vi "TransistorOnOff.vi"() -> ()   [LabVIEW 2014]
uses:
  <vilib>/DAQmx/create/channels.llb/DAQmx Create Channel (AI-Voltage-Basic).vi
  <vilib>/DAQmx/create/channels.llb/DAQmx Create Channel (DO-Digital Output).vi
  <vilib>/DAQmx/read.llb/DAQmx Read (Analog DBL 1Chan 1Samp).vi
  <vilib>/DAQmx/write.llb/DAQmx Write (Digital Bool 1Line 1Point).vi
panel:
  out "?":bool
  in  "VREF \nVoltage Measured from unheated":dbl
  out "Analog Voltage":dbl
  in  "Ambient Temperature (C)":dbl=22.0
  in  "Low Setpoint (C)":dbl=30.0
  in  "Hi Setpoint (C)":dbl=33.0
  in  "dt (ms)":dbl=0.5 format="%#_13g"
  out "Sample Temp":dbl
  out "?":dbl(graph)
  in  "?":bool
  out "Heater Output":dbl(slide) scale=0.0..1.0
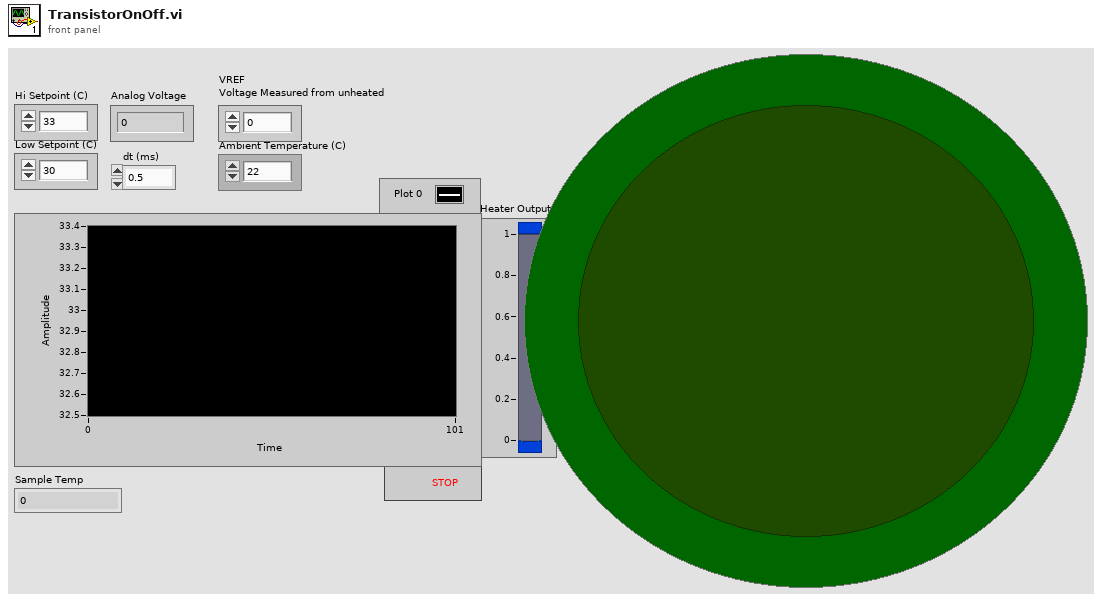
[diagram p1: front panel]
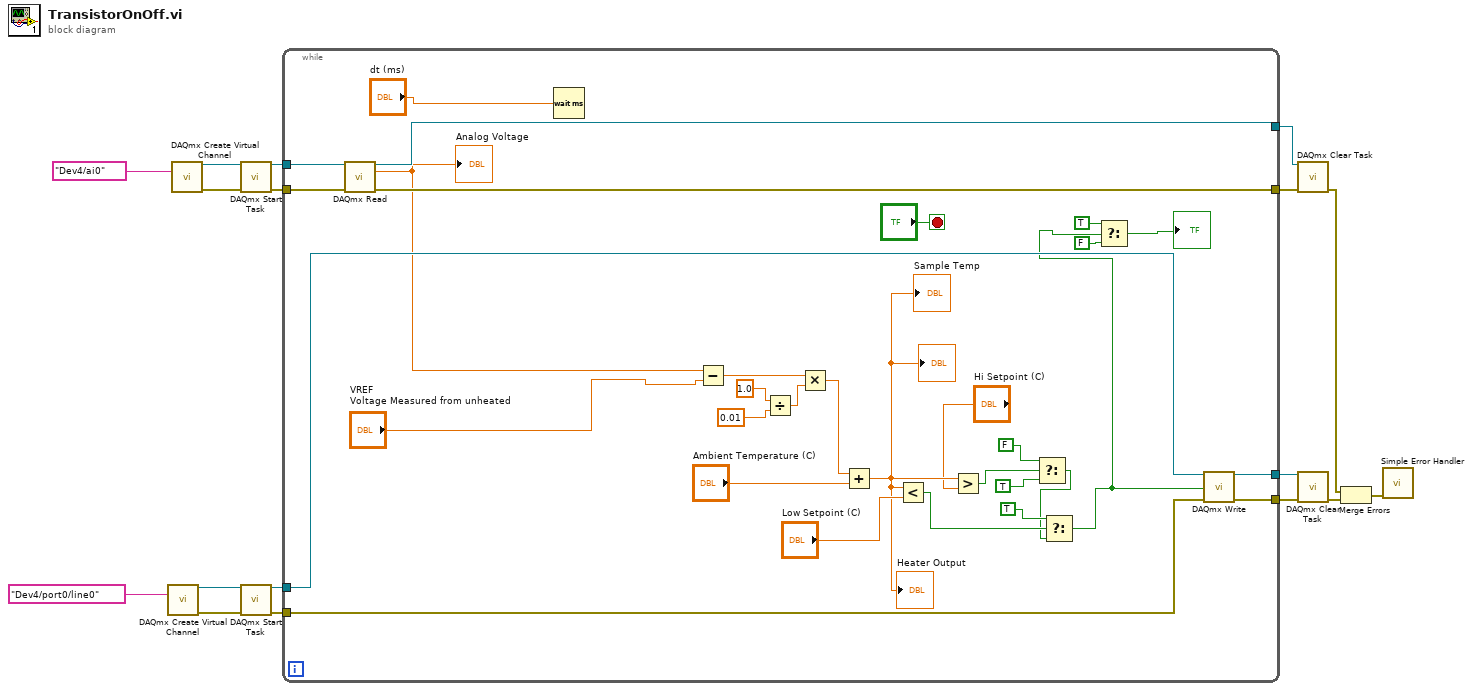
[diagram p0: block diagram]
diagram:
  n1 = call-poly <vilib>:"DAQmx Create Virtual Channel.vi"("lines"=tag "Dev4/port0/line0") -> ("task out"=w10:refnum<k21>, "error out"=w9:errorcluster)  [unwired: 13 in]
  n2 = call-poly <vilib>:"DAQmx Create Virtual Channel.vi"("physical channels"=tag "Dev4/ai0") -> ("task out"=w16:refnum<k21>, "error out"=w17:errorcluster)  [unwired: 13 in]
  n3 = call <vilib>:"DAQmx Start Task.vi"("task/channels in"=w16, "error in"=w17) -> ("task out"=w14:refnum<k21>, "error out"=w13:errorcluster)  [unwired: 12 in]
  n4 = call <vilib>:"DAQmx Start Task.vi"("task/channels in"=w10, "error in"=w9) -> ("task out"=w8:refnum<k21>, "error out"=w7:errorcluster)  [unwired: 12 in]
  n5 = while {
    tunnel: w14 -> [w47]
    tunnel: w13 -> [w46]
    tunnel: [w45] -> w12
    tunnel: [w44] -> w11
    tunnel: w8 -> [w37]
    tunnel: w7 -> [w36]
    tunnel: [w35] -> w6
    tunnel: [w34] -> w5
    stop <- "?" stop-if-true
    n6 = call-poly <vilib>:"DAQmx Read.vi"("task/channels in"=w47, "error in"=w46) -> ("task out"=w45:refnum<k21>, "data"=w31:dbl, "error out"=w44:errorcluster)  [unwired: 11 in]
    "Analog Voltage" <- w31
    n7 = Wait (ms)(milliseconds to wait="dt (ms)") -> ()  [unwired: 1 out]
    n8 = Subtract(x=w31, y="VREF \nVoltage Measured from unheated") -> (x-y=w39:dbl)
    n9 = Divide(x=1.0, y=0.01) -> (x/y=w42:dbl)
    n10 = Multiply(x=w39, y=w42) -> (x*y=w38:dbl)
    n11 = Add(x=w38, y="Ambient Temperature (C)") -> (x+y=w30:dbl)
    "Heater Output" <- w30
    "?" <- w30
    "Sample Temp" <- w30
    n12 = Less?(x=w30, y="Low Setpoint (C)") -> (x < y?=w23:bool)
    n13 = Greater?(x=w30, y="Hi Setpoint (C)") -> (0:w26:bool)
    n14 = Select(t=FALSE, s=w26, f=TRUE) -> (s? t:f=w21:bool)
    n15 = Select(t=TRUE, s=w23, f=w21) -> (s? t:f=w20:bool)
    n16 = Select(t=TRUE, s=w20, f=FALSE) -> (s? t:f=→"?":bool)
    n17 = call-poly <vilib>:"DAQmx Write.vi"("task/channels in"=w37, "data"=w20, "error in"=w36) -> ("task out"=w34:refnum<k21>, "error out"=w35:errorcluster)  [unwired: 10 in, 1 out]
  }
  n18 = call <vilib>:"DAQmx Clear Task.vi"("task in"=w12, "error in"=w11) -> ("error out"=w4:errorcluster)  [unwired: 13 in]
  n19 = call <vilib>:"DAQmx Clear Task.vi"("task in"=w5, "error in"=w6) -> ("error out"=w3:errorcluster)  [unwired: 13 in]
  n20 = Merge Errors(w4, w3) -> (w2:errorcluster)
  n21 = call <vilib>:"Simple Error Handler.vi"("error in (no error)"=w2) -> ()  [unwired: 4 in, 5 out]
